vi "Meas Proc QWTB Multicore Start Servers.vi"(8 "error in":errorcluster, 11 "session in":T1={"adc"={"niScope"={"channel cfg"=[], "sessions"=[], "multi cards"=FALSE, "channels"=0, "type"=enum."n/a", "memory [B/chn]"=0, "ext. clock [Hz]"=0.0, "samples count"=0, "use streaming"=FALSE, "proc setup"={"packet size [smpl]"=0, "current timeout [s]"=0.0, "blk2blk timeout [s]"=0.0, "event time"=timestamp(0 s since 1904-01-01), "temp sampl T [s]"=0.0, "data queue"=refnum, "stop notifier"=refnum, "proc ref"=refnum}, "sample width [B]"=0, "ranges [V]"=[], "trigger setup"={"coupling"=1, "level [V]"=0.0, "slope"=0, "mode"=enum."Immediate"}, "fs [Hz]"=0.0, "bitres [bit]"=0, "clock source"=enum."VAL_NO_SOURCE"}, "3458A"={"channels"=[], "sync unit"={"VISA"="", "type"=enum."Picotest U6200A"}, "awg unit"={"type"=enum."Agilent 331xxA to 332xxA", "VISA"="", "enable 10MHz ref"=FALSE}, "sync mode"=enum."MASTER-SLAVE, MASTER clocked by TIMER", "streaming mode"=FALSE, "idn mode"=enum."Auto", "sampling mode"=enum."DCV", "Ts [s]"=0.0, "sample memory [B]"=0, "proc setup"={"channel id"=0, "packet size [smpl]"=0, "current timeout [s]"=0.0, "blk2blk timeout [s]"=0.0, "event time"=timestamp(0 s since 1904-01-01), "stop notifier"=refnum, "data queues"=[], "proc refs"=[], "bus semaphore"=refnum}, "sample size [B]"=0, "sample count"=0, "aux data"={"channel id"=0, "valid?"=[], "gain [V]"=[], "timestamp [s]"=[], "Ts [s]"=0.0, "abs timestamp"=timestamp(0 s since 1904-01-01), "t [deg C]"=[], "multiplex timestamp [s]"=-1.0, "only multiplex?"=FALSE, "multiplex smpl offset"=0}, "ranges [V]"=[], "aperture [s]"=0.0, "LEVEL trigger"={"edge"=enum."POS", "level [V]"=0.0, "coupling"=enum."DC"}, "trigger mode"=enum."AUTO", "measure temp.?"=FALSE, "disp mesages"=[], "shared bus?"=FALSE, "disable display?"=FALSE, "aper mode"=enum."Manual", "aper rules"=[], "multiplex"={"cycles"=0, "delay [s]"=0.0, "enabled"=FALSE, "overhead [s]"=1.0, "tot smpls"=0}}, "dsdll"={"dsdll"={"dsdll path"=path "", "dsdll handle"=[], "output devices"=[], "capture devices"=[]}, "channels"=0, "device id"=0, "channel idns"=[], "proc setup"={"packet size [smpl]"=0, "current timeout [s]"=0.0, "blk2blk timeout [s]"=0.0, "event time"=timestamp(0 s since 1904-01-01), "data queue"=refnum, "stop notifier"=refnum, "proc ref"=refnum}, "samples count"=0, "fs [Hz]"=0.0}, "type"=enum."niScope", "channel idn str"=[], "aux instr idn str"=[], "modified?"=FALSE, "simadc"={"channels"=[], "range [V]"=0.0, "Ts step [s]"=0.0, "time [s]"=0.0, "fs [Hz]"=0.0, "count"=0, "smpl offset"=0, "set count"=0, "bit res"=0}, "force rst?"=FALSE, "exit mode"=enum."Immediate reset", "exit dly"=0.0, "exit tmr"=timestamp(0 s since 1904-01-01), "busy?"=FALSE, "accessed?"=FALSE, "multiplex"={"Type"=enum."Dummy", "gen com ssn"={"visa"="", "primary"=enum."None", "secondary"=enum."None", "channels"=[]}, "delay before [s]"=0.0, "delay post [s]"=0.0, "sequence"=[], "enabled"=FALSE, "ref timestamp [s]"=0.0, "idn string"="", "dev niScope"="", "niScope idx"=0}}, "sequence"=[], "sequence setup"={"group setups"=[], "average cycles"=0, "range mode"=enum."Keep defaults", "fs mode"=enum."Frequency", "rng even"=0.0, "rng odd"=0.0, "folder"=path "", "name base"="", "meas id"=0, "settle [s]"=0.0, "comment"=""}, "golpi"=refnum, "processing setup"={"mode"=enum."Raw", "call after avgs?"=FALSE, "calculate?"=FALSE, "raw mode"={"command"="", "result mode"=enum."Display console output (only Octave)", "res variable"=""}, "QWTB"={"QWTB path"=path "", "alg filter path"="", "alg ids"=[], "alg parameters"=[], "parsed parameters"=[], "selected alg id"="", "selected unc mode"=enum."None", "qwtb mcc"=100, "qwtb timeout"=90, "qwtb covg"=95.0, "qwtb ofs"=0, "qwtb lim data"=0, "multicore"={"jobs folder"=path "", "cores"=0, "max jobs"=0, "mode"=enum."Singlecore"}, "unc once?"=FALSE, "qwtb tstemp"=enum."Enabled (default)", "octave reset"=FALSE}}, "corrections"={"transducers"={"channels"=[], "last path"=path ""}, "digitizer"={"last path"=path "", "channel paths"=[], "channel idns"=[], "correction name"="", "channel names"=[], "folders to copy"=[], "channel valid"=[], "correction path"=path "", "correction rel path"="", "rel folders to copy"=[]}}, "assist cfg"={"P"=0, "Q"=0, "rel shift"=0.0, "ref freq"=0.0, "min fs"=0.0, "max fs tol"=0.0, "min int"=0.0, "max int"=0.0, "max err"=0.0, "max timeout"=0.0}} {"corrections"."transducers"."channels"."Phase index" min=1 step=1; "adc"."3458A"."channels"."Range [Vpk]" min=0.0; "adc"."niScope"."trigger setup"."level [V]" format="%.2f"; "adc"."niScope"."trigger setup"."coupling" items=["AC"=0, "DC"=1, "HF Reject"=3, "LF Reject"=4, "AC Plus HF Reject"=1001]; "adc"."niScope"."channel cfg"."Range [Vpk]" min=0.0; "adc"."niScope"."channel cfg"."Channel" min=0}) -> (0 "error out":errorcluster, 3 "session out":T1={"adc"={"niScope"={"channel cfg"=[], "sessions"=[], "multi cards"=FALSE, "channels"=0, "type"=enum."n/a", "memory [B/chn]"=0, "ext. clock [Hz]"=0.0, "samples count"=0, "use streaming"=FALSE, "proc setup"={"packet size [smpl]"=0, "current timeout [s]"=0.0, "blk2blk timeout [s]"=0.0, "event time"=timestamp(0 s since 1904-01-01), "temp sampl T [s]"=0.0, "data queue"=refnum, "stop notifier"=refnum, "proc ref"=refnum}, "sample width [B]"=0, "ranges [V]"=[], "trigger setup"={"coupling"=1, "level [V]"=0.0, "slope"=0, "mode"=enum."Immediate"}, "fs [Hz]"=0.0, "bitres [bit]"=0, "clock source"=enum."VAL_NO_SOURCE"}, "3458A"={"channels"=[], "sync unit"={"VISA"="", "type"=enum."Picotest U6200A"}, "awg unit"={"type"=enum."Agilent 331xxA to 332xxA", "VISA"="", "enable 10MHz ref"=FALSE}, "sync mode"=enum."MASTER-SLAVE, MASTER clocked by TIMER", "streaming mode"=FALSE, "idn mode"=enum."Auto", "sampling mode"=enum."DCV", "Ts [s]"=0.0, "sample memory [B]"=0, "proc setup"={"channel id"=0, "packet size [smpl]"=0, "current timeout [s]"=0.0, "blk2blk timeout [s]"=0.0, "event time"=timestamp(0 s since 1904-01-01), "stop notifier"=refnum, "data queues"=[], "proc refs"=[], "bus semaphore"=refnum}, "sample size [B]"=0, "sample count"=0, "aux data"={"channel id"=0, "valid?"=[], "gain [V]"=[], "timestamp [s]"=[], "Ts [s]"=0.0, "abs timestamp"=timestamp(0 s since 1904-01-01), "t [deg C]"=[], "multiplex timestamp [s]"=-1.0, "only multiplex?"=FALSE, "multiplex smpl offset"=0}, "ranges [V]"=[], "aperture [s]"=0.0, "LEVEL trigger"={"edge"=enum."POS", "level [V]"=0.0, "coupling"=enum."DC"}, "trigger mode"=enum."AUTO", "measure temp.?"=FALSE, "disp mesages"=[], "shared bus?"=FALSE, "disable display?"=FALSE, "aper mode"=enum."Manual", "aper rules"=[], "multiplex"={"cycles"=0, "delay [s]"=0.0, "enabled"=FALSE, "overhead [s]"=1.0, "tot smpls"=0}}, "dsdll"={"dsdll"={"dsdll path"=path "", "dsdll handle"=[], "output devices"=[], "capture devices"=[]}, "channels"=0, "device id"=0, "channel idns"=[], "proc setup"={"packet size [smpl]"=0, "current timeout [s]"=0.0, "blk2blk timeout [s]"=0.0, "event time"=timestamp(0 s since 1904-01-01), "data queue"=refnum, "stop notifier"=refnum, "proc ref"=refnum}, "samples count"=0, "fs [Hz]"=0.0}, "type"=enum."niScope", "channel idn str"=[], "aux instr idn str"=[], "modified?"=FALSE, "simadc"={"channels"=[], "range [V]"=0.0, "Ts step [s]"=0.0, "time [s]"=0.0, "fs [Hz]"=0.0, "count"=0, "smpl offset"=0, "set count"=0, "bit res"=0}, "force rst?"=FALSE, "exit mode"=enum."Immediate reset", "exit dly"=0.0, "exit tmr"=timestamp(0 s since 1904-01-01), "busy?"=FALSE, "accessed?"=FALSE, "multiplex"={"Type"=enum."Dummy", "gen com ssn"={"visa"="", "primary"=enum."None", "secondary"=enum."None", "channels"=[]}, "delay before [s]"=0.0, "delay post [s]"=0.0, "sequence"=[], "enabled"=FALSE, "ref timestamp [s]"=0.0, "idn string"="", "dev niScope"="", "niScope idx"=0}}, "sequence"=[], "sequence setup"={"group setups"=[], "average cycles"=0, "range mode"=enum."Keep defaults", "fs mode"=enum."Frequency", "rng even"=0.0, "rng odd"=0.0, "folder"=path "", "name base"="", "meas id"=0, "settle [s]"=0.0, "comment"=""}, "golpi"=refnum, "processing setup"={"mode"=enum."Raw", "call after avgs?"=FALSE, "calculate?"=FALSE, "raw mode"={"command"="", "result mode"=enum."Display console output (only Octave)", "res variable"=""}, "QWTB"={"QWTB path"=path "", "alg filter path"="", "alg ids"=[], "alg parameters"=[], "parsed parameters"=[], "selected alg id"="", "selected unc mode"=enum."None", "qwtb mcc"=100, "qwtb timeout"=90, "qwtb covg"=95.0, "qwtb ofs"=0, "qwtb lim data"=0, "multicore"={"jobs folder"=path "", "cores"=0, "max jobs"=0, "mode"=enum."Singlecore"}, "unc once?"=FALSE, "qwtb tstemp"=enum."Enabled (default)", "octave reset"=FALSE}}, "corrections"={"transducers"={"channels"=[], "last path"=path ""}, "digitizer"={"last path"=path "", "channel paths"=[], "channel idns"=[], "correction name"="", "channel names"=[], "folders to copy"=[], "channel valid"=[], "correction path"=path "", "correction rel path"="", "rel folders to copy"=[]}}, "assist cfg"={"P"=0, "Q"=0, "rel shift"=0.0, "ref freq"=0.0, "min fs"=0.0, "max fs tol"=0.0, "min int"=0.0, "max int"=0.0, "max err"=0.0, "max timeout"=0.0}} {"corrections"."transducers"."channels"."Phase index" min=1 step=1; "adc"."3458A"."channels"."Range [Vpk]" min=0.0; "adc"."niScope"."trigger setup"."level [V]" format="%.2f"; "adc"."niScope"."trigger setup"."coupling" items=["AC"=0, "DC"=1, "HF Reject"=3, "LF Reject"=4, "AC Plus HF Reject"=1001]; "adc"."niScope"."channel cfg"."Range [Vpk]" min=0.0; "adc"."niScope"."channel cfg"."Channel" min=0})   [LabVIEW 2013]
doc: "Start multistation mode servers."
uses:
  Meas Session.ctl
  adc/ADC Session.ctl
  drivers/niScope/niScope Session.ctl
  drivers/niScope/niScope Virtual Channel Config.ctl
  drivers/niScope/niScope Virtual Channel Mode.ctl
  drivers/niScope/niScope Virtual Channel Input Z.ctl
  drivers/niScope/niScope Virtual Channel Coupling.ctl
  drivers/niScope/niScope Type.ctl
  drivers/niScope/niScope Digitizing Process Options.ctl
  drivers/niScope/niScope Data Packet.ctl
  drivers/niScope/niScope Trigger Setup.ctl
  <instrlib>/niScope/Controls/niScope trigger coupling.ctl
  <instrlib>/niScope/Controls/niScope trigger slope.ctl
  drivers/niScope/niScope Reference Clock.ctl
  drivers/DMM/3458A Digitizer Session.ctl
  drivers/DMM/3458A Virtual Channel Config.ctl
  drivers/Counter/Counter Session.ctl
  drivers/Counter/Counter Type.ctl
  drivers/AWG/AWG Session.ctl
  drivers/AWG/AWG Type.ctl
  drivers/DMM/3458A Sync Mode.ctl
  drivers/DMM/3458A Idn Mode.ctl
  drivers/DMM/3458A Digitizing Low Levels/Configure/Sampling Mode.ctl
  drivers/DMM/3458A Digitizing Process Options.ctl
  drivers/DMM/3458A Data Packet.ctl
  drivers/DMM/3458A Aux Record Data.ctl
  drivers/DMM/3458A Digitizing Low Levels/Configure/Level Setup.ctl
  drivers/DMM/3458A Digitizing Low Levels/Configure/First Sample Trigger.ctl
  drivers/DMM/3458A Aperture Selection Mode.ctl
  drivers/DMM/3458A Multiplexing Config.ctl
  drivers/dsdll/DSDLL Session.ctl
  drivers/dsdll/dsdll.lvlibp/dsdll_instance.ctl
  drivers/dsdll/dsdll.lvlibp/dsdll_device_record.ctl
  drivers/dsdll/DSDLL Process Config.ctl
  drivers/dsdll/DSDLL Data Packet.ctl
  adc/ADC Type.ctl
  drivers/simulated_adc/SimAdc Config.ctl
  drivers/simulated_adc/SimAdc Channel Cfg.ctl
  adc/ADC On Close Action.ctl
  adc/Multiplexer/MPX Session.ctl
  adc/Multiplexer/MPX Type.ctl
  drivers/Multiplexers/Generic COM/GCOMM Session.ctl
  drivers/Multiplexers/Generic COM/GCOMM Signal.ctl
  drivers/Multiplexers/Generic COM/GCOMM Virtual Channel.ctl
  drivers/Multiplexers/Generic COM/GCOMM Logic State.ctl
  Meas Sequence Item.ctl
  Meas Sampling Configuration.ctl
  adc/ADC Trig Config.ctl
  adc/ADC Trig Mode Source.ctl
  adc/ADC Trig Coupling.ctl
  adc/ADC Trig Slope.ctl
  Meas Proc QWTB Algorithm Parameter Data.ctl
  Meas Sequence Configuration.ctl
  Meas Range Mode.ctl
  Meas Sampling Rate Mode.ctl
  octave/golpi/mpc/golpi_session_ref.ctl
  octave/golpi/mpc/golpi_session.ctl
  octave/golpi/GOLPI Library.lvlibp/Public/GOLPI reference Type Def.ctl
  octave/golpi/GOLPI Library.lvlibp/LV Process source distribution/Pipe Handle.ctl
  Meas Process Config.ctl
  Meas Process Mode.ctl
  Meas Process Raw Config.ctl
  Meas Process Raw Result Mode.ctl
  Meas Proc QWTB Setup.ctl
  Meas Proc QWTB Uncertainty Mode.ctl
  Meas Proc QWTB Multicore Setup.ctl
  Meas Proc QWTB Multicore Type.ctl
  Meas Process Time Stamp Mode.ctl
  Corrections/Corr Setup.ctl
  Corrections/Corr Tranducer Item.ctl
  Corrections/Corr Digitizers.ctl
  Assist/Assist Panel Setup.ctl
  <vilib>/Utility/error.llb/Error Cluster From Error Code.vi
  <vilib>/ErrorRing/Error Ring.xnode
  octave/golpi/mpc/GOLPI Multi Process.lvlib
  octave/golpi/GOLPI Library.lvlibp
  drivers/niScope/niScope Virtual Digitizer.lvlib
  drivers/DMM/3458A Virtual Digitizer.lvlib
  drivers/Counter/Counter.lvlib
  drivers/AWG/AWG.lvlib
  drivers/DMM/3458A Digitizing Low Levels/3458A Digitizing Low Levels.lvlib
  drivers/dsdll/dsdll.lvlibp
  drivers/dsdll/DSDLL Virtual Digitizer.lvlib
  octave/golpi/GOLPI Library.lvlibp/LV Process source distribution/LV Process library.lvlib
panel:
  # "ADC:"
  # "ADC:"
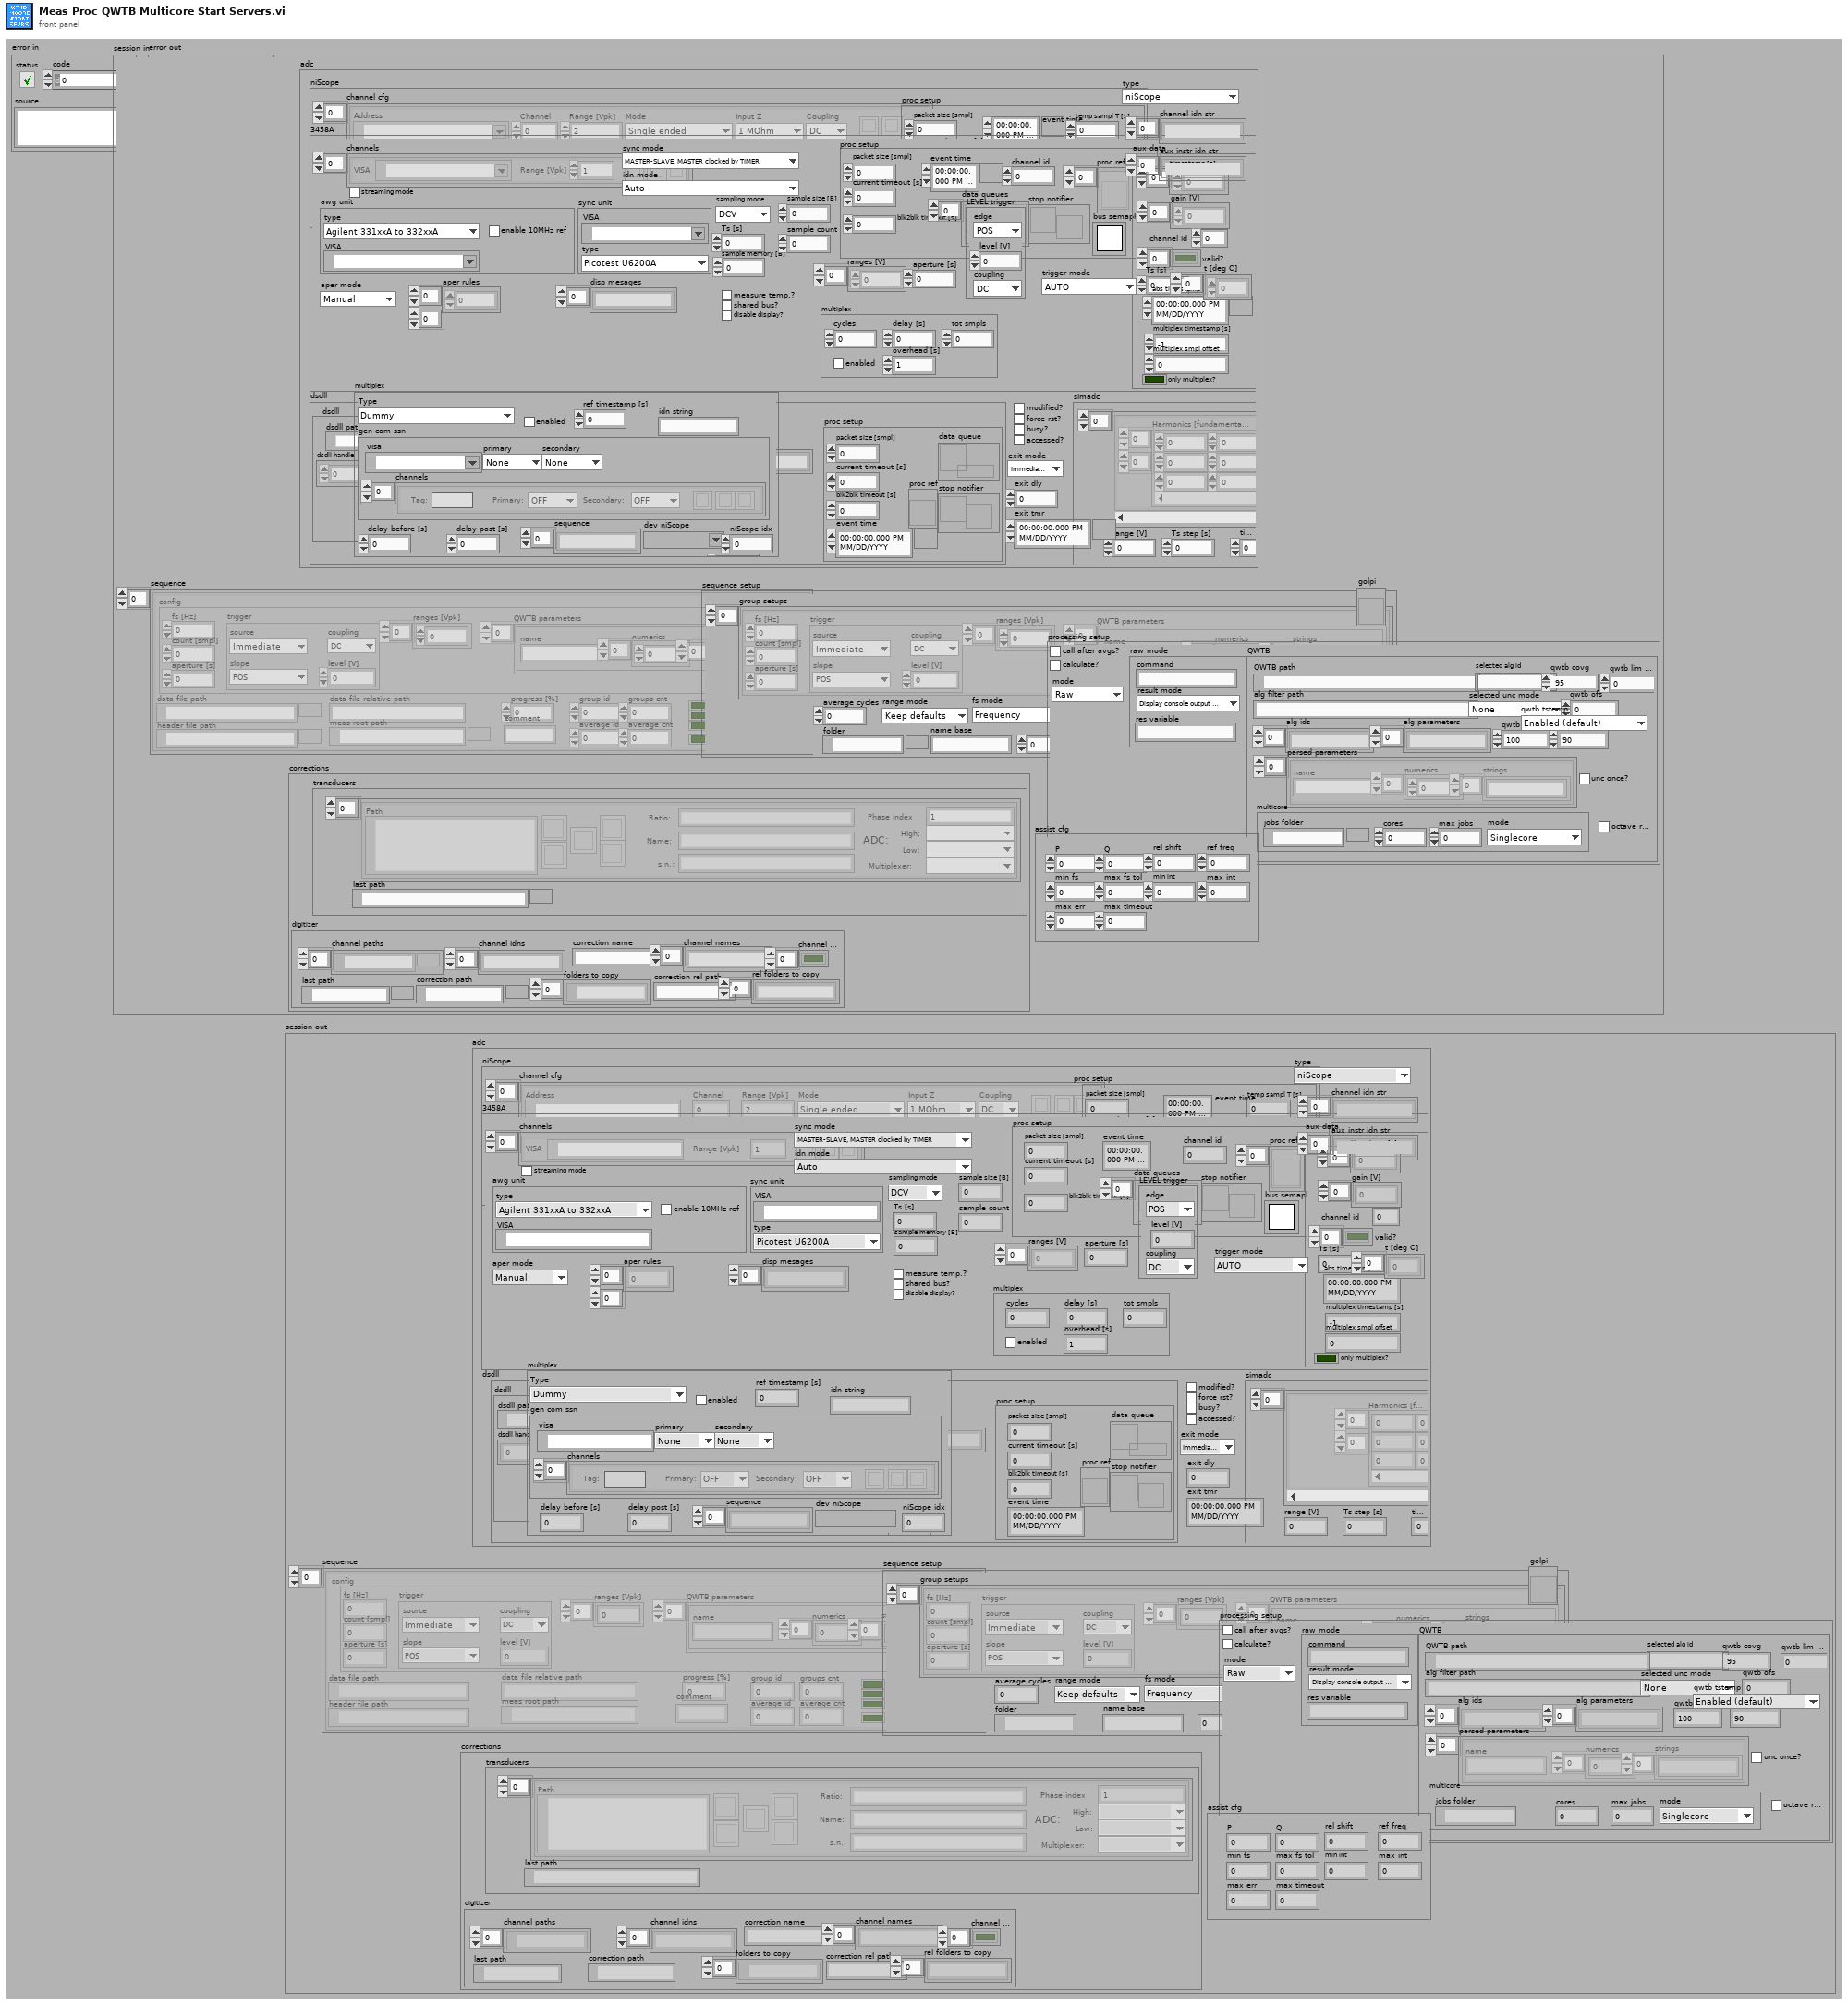
[diagram p1: front panel]
types:
  T1 = typedef "Meas Session.ctl" = cluster{"adc":T2, "sequence":T44[], "sequence setup":T51, "golpi":T54, "processing setup":T55, "corrections":T64, "assist cfg":T67}
  T2 = typedef "ADC Session.ctl" = cluster{"niScope":T3, "3458A":T14, "dsdll":T30, "type":T34, "channel idn str":string[], "aux instr idn str":string[], "modified?":bool, "simadc":T35, "force rst?":bool, "exit mode":T37, "exit dly":dbl, "exit tmr":timestamp, "busy?":bool, "accessed?":bool, "multiplex":T38}
  T3 = typedef "niScope Virtual Digitizer.lvlib/niScope Session.ctl" = cluster{"channel cfg":T4[], "sessions":refnum<k20>[], "multi cards":bool, "channels":i32, "type":T8, "memory [B/chn]":i32, "ext. clock [Hz]":dbl, "samples count":i64, "use streaming":bool, "proc setup":T9, "sample width [B]":i32, "ranges [V]":dbl[], "trigger setup":T10, "fs [Hz]":dbl, "bitres [bit]":i32, "clock source":T13}
  T4 = typedef "niScope Virtual Digitizer.lvlib/niScope Virtual Channel Config.ctl" = cluster{"Address":refnum<k15>, "Channel":i32, "Mode":T5, "Input Z":T6, "Coupling":T7, "Range [Vpk]":dbl, "btn clr":bool, "btn up":bool, "btn down":bool}
  T5 = typedef "niScope Virtual Digitizer.lvlib/niScope Virtual Channel Mode.ctl" = enum16{"Single ended", "Unbal. differential", "Differential"}
  T6 = typedef "niScope Virtual Digitizer.lvlib/niScope Virtual Channel Input Z.ctl" = enum16{"1 MOhm", "50 Ohm"}
  T7 = typedef "niScope Virtual Digitizer.lvlib/niScope Virtual Channel Coupling.ctl" = enum16{"AC", "DC", "GND"}
  T8 = typedef "niScope Virtual Digitizer.lvlib/niScope Type.ctl" = enum16{"n/a", "5922"}
  T9 = typedef "niScope Virtual Digitizer.lvlib/niScope Digitizing Process Options.ctl" = cluster{"packet size [smpl]":i64, "current timeout [s]":dbl, "blk2blk timeout [s]":dbl, "event time":timestamp, "temp sampl T [s]":dbl, "data queue":refnum<queue>, "stop notifier":refnum<notifier>, "proc ref":refnum<vi>}
  T10 = typedef "niScope Virtual Digitizer.lvlib/niScope Trigger Setup.ctl" = cluster{"coupling":T11, "level [V]":dbl, "slope":T12, "mode":enum16{"Immediate", "External", "Level"}}
  T11 = typedef "niScope trigger coupling.ctl" = u16
  T12 = typedef "niScope trigger slope.ctl" = i32
  T13 = typedef "niScope Virtual Digitizer.lvlib/niScope Reference Clock.ctl" = enum16{"VAL_NO_SOURCE", "VAL_CLK_IN", "VAL_PXI_CLOCK", "VAL_EXTERNAL"}
  T14 = typedef "3458A Virtual Digitizer.lvlib/3458A Digitizer Session.ctl" = cluster{"channels":T15[], "sync unit":T16, "awg unit":T18, "sync mode":T20, "streaming mode":bool, "idn mode":T21, "sampling mode":T22, "Ts [s]":dbl, "sample memory [B]":i32, "proc setup":T23, "sample size [B]":i32, "sample count":i32, "aux data":T25, "ranges [V]":dbl[], "aperture [s]":dbl, "LEVEL trigger":T26, "trigger mode":T27, "measure temp.?":bool, "disp mesages":string[], "shared bus?":bool, "disable display?":bool, "aper mode":T28, "aper rules":dbl[][], "multiplex":T29}
  T15 = typedef "3458A Virtual Digitizer.lvlib/3458A Virtual Channel Config.ctl" = cluster{"VISA":refnum<visa-resource-name>, "Range [Vpk]":dbl, "btn clr":bool, "btn up":bool, "btn down":bool}
  T16 = typedef "Counter.lvlib/Counter Session.ctl" = cluster{"VISA":refnum<visa-resource-name>, "type":T17}
  T17 = typedef "Counter.lvlib/Counter Type.ctl" = enum16{"Picotest U6200A", "dummy"}
  T18 = typedef "AWG.lvlib/AWG Session.ctl" = cluster{"type":T19, "VISA":refnum<visa-resource-name>, "enable 10MHz ref":bool}
  T19 = typedef "AWG.lvlib/AWG Type.ctl" = enum16{"Agilent 331xxA to 332xxA", "Agilent 335xxA to 336xxA", "Tektronix AFG3101C", "dummy"}
  T20 = typedef "3458A Virtual Digitizer.lvlib/3458A Sync Mode.ctl" = enum16{"MASTER-SLAVE, MASTER clocked by TIMER", "MASTER-SLAVE, MASTER clocked by AWG", "ALL clocked by AWG", "MASTER-SLAVE, ALL clocked by TIMER", "ALL clocked by AWG with DFLL"}
  T21 = typedef "3458A Virtual Digitizer.lvlib/3458A Idn Mode.ctl" = enum16{"Auto", "Sequential (chn A, chn B, ...)", "From calibration string"}
  T22 = typedef "3458A Virtual Digitizer.lvlib/3458A Digitizing Low Levels.lvlib/Sampling Mode.ctl" = enum16{"DCV", "DSDC", "DSAC"}
  T23 = typedef "3458A Virtual Digitizer.lvlib/3458A Digitizing Process Options.ctl" = cluster{"channel id":i32, "packet size [smpl]":i32, "current timeout [s]":dbl, "blk2blk timeout [s]":dbl, "event time":timestamp, "stop notifier":refnum<notifier>, "data queues":refnum<queue>[], "proc refs":refnum<vi>[], "bus semaphore":T24}
  T24 = typedef "Semaphore RefNum" = refnum<k1>
  T25 = typedef "3458A Virtual Digitizer.lvlib/3458A Aux Record Data.ctl" = cluster{"channel id":i32, "valid?":bool[], "gain [V]":dbl[], "timestamp [s]":dbl[], "Ts [s]":dbl, "abs timestamp":timestamp, "t [deg C]":dbl[], "multiplex timestamp [s]":dbl, "only multiplex?":bool, "multiplex smpl offset":i64}
  T26 = typedef "3458A Virtual Digitizer.lvlib/3458A Digitizing Low Levels.lvlib/Level Setup.ctl" = cluster{"edge":enum16{"POS", "NEG"}, "level [V]":dbl, "coupling":enum16{"DC", "AC"}}
  T27 = typedef "3458A Virtual Digitizer.lvlib/3458A Digitizing Low Levels.lvlib/First Sample Trigger.ctl" = enum16{"AUTO", "EXT", "SYN", "SGL", "HOLD", "LEVEL"}
  T28 = typedef "3458A Virtual Digitizer.lvlib/3458A Aperture Selection Mode.ctl" = enum16{"Manual", "Maximum", "Table"}
  T29 = typedef "3458A Multiplexing Config.ctl" = cluster{"cycles":i32, "delay [s]":dbl, "enabled":bool, "overhead [s]":dbl, "tot smpls":i64}
  T30 = typedef "DSDLL Virtual Digitizer.lvlib/DSDLL Session.ctl" = cluster{"dsdll":T31, "channels":i32, "device id":i32, "channel idns":string[], "proc setup":T33, "samples count":i32, "fs [Hz]":dbl}
  T31 = typedef "dsdll.lvlibp/dsdll_instance.ctl" = cluster{"dsdll path":path, "dsdll handle":u8[], "output devices":T32[], "capture devices":T32[]}
  T32 = typedef "dsdll.lvlibp/dsdll_device_record.ctl" = cluster{"guid":u8[], "name":string}
  T33 = typedef "DSDLL Virtual Digitizer.lvlib/DSDLL Process Config.ctl" = cluster{"packet size [smpl]":i32, "current timeout [s]":dbl, "blk2blk timeout [s]":dbl, "event time":timestamp, "data queue":refnum<queue>, "stop notifier":refnum<notifier>, "proc ref":refnum<vi>}
  T34 = typedef "ADC Type.ctl" = enum16{"niScope", "3458A", "DirectSound DLL", "dummy"}
  T35 = typedef "SimAdc Config.ctl" = cluster{"channels":T36[], "range [V]":dbl, "Ts step [s]":dbl, "time [s]":dbl, "fs [Hz]":dbl, "count":i64, "smpl offset":i64, "set count":i64, "bit res":i32}
  T36 = typedef "SimAdc Channel Cfg.ctl" = cluster{"harmonics":dbl[][], "btn clear":bool, "noise":dbl, "fundamental [Hz]":dbl}
  T37 = typedef "ADC On Close Action.ctl" = enum16{"Immediate reset", "Delayed reset"}
  T38 = typedef "MPX Session.ctl" = cluster{"Type":T39, "gen com ssn":T40, "delay before [s]":dbl, "delay post [s]":dbl, "sequence":string[], "enabled":bool, "ref timestamp [s]":dbl, "idn string":string, "dev niScope":refnum<k15>, "niScope idx":i32}
  T39 = typedef "MPX Type.ctl" = enum16{"Dummy", "Generic - COM port", "Generic - niScope PFI"}
  T40 = typedef "GCOMM Session.ctl" = cluster{"visa":refnum<visa-resource-name>, "primary":T41, "secondary":T41, "channels":T42[]}
  T41 = typedef "GCOMM Signal.ctl" = enum16{"None", "DTR", "RTS"}
  T42 = typedef "GCOMM Virtual Channel.ctl" = cluster{"Primary:":T43, "Secondary:":T43, "btn clr":bool, "btn up":bool, "btn down":bool, "Tag:":string}
  T43 = typedef "GCOMM Logic State.ctl" = enum16{"OFF", "ON"}
  T44 = typedef "Meas Sequence Item.ctl" = cluster{"config":T45, "data file path":path, "header file path":path, "group id":i32, "average id":i32, "group done?":bool, "adc modified?":bool, "source modified?":bool, "progress [%]":dbl, "groups cnt":i32, "average cnt":i32, "data file relative path":string, "meas root path":path, "calculate?":bool, "comment":string}
  T45 = typedef "Meas Sampling Configuration.ctl" = cluster{"fs [Hz]":dbl, "count [smpl]":i64, "aperture [s]":dbl, "trigger":T46, "ranges [Vpk]":dbl[], "QWTB parameters":T50[]}
  T46 = typedef "ADC Trig Config.ctl" = cluster{"source":T47, "level [V]":dbl, "coupling":T48, "slope":T49}
  T47 = typedef "ADC Trig Mode Source.ctl" = enum16{"Immediate", "External", "Level"}
  T48 = typedef "ADC Trig Coupling.ctl" = enum16{"DC", "AC"}
  T49 = typedef "ADC Trig Slope.ctl" = enum16{"POS", "NEG"}
  T50 = typedef "Meas Proc QWTB Algorithm Parameter Data.ctl" = cluster{"name":string, "numerics":dbl[], "strings":string[]}
  T51 = typedef "Meas Sequence Configuration.ctl" = cluster{"group setups":T45[], "average cycles":i32, "range mode":T52, "fs mode":T53, "rng even":dbl, "rng odd":dbl, "folder":path, "name base":string, "meas id":i32, "settle [s]":dbl, "comment":string}
  T52 = typedef "Meas Range Mode.ctl" = enum16{"Keep defaults", "Set All channels", "Set Odd and Even channels"}
  T53 = typedef "Meas Sampling Rate Mode.ctl" = enum16{"Frequency", "Period"}
  T54 = typedef "GOLPI Multi Process.lvlib/golpi_session_ref.ctl" = refnum<vi>
  T55 = typedef "Meas Process Config.ctl" = cluster{"mode":T56, "call after avgs?":bool, "calculate?":bool, "raw mode":T57, "QWTB":T59}
  T56 = typedef "Meas Process Mode.ctl" = enum16{"Raw", "QWTB"}
  T57 = typedef "Meas Process Raw Config.ctl" = cluster{"command":string, "result mode":T58, "res variable":string}
  T58 = typedef "Meas Process Raw Result Mode.ctl" = enum16{"Display console output (only Octave)", "Display string variable", "Display result file %respath%"}
  T59 = typedef "Meas Proc QWTB Setup.ctl" = cluster{"QWTB path":path, "alg filter path":string, "alg ids":string[], "alg parameters":string[], "parsed parameters":T50[], "selected alg id":string, "selected unc mode":T60, "qwtb mcc":i32, "qwtb timeout":i32, "qwtb covg":dbl, "qwtb ofs":i64, "qwtb lim data":i64, "multicore":T61, "unc once?":bool, "qwtb tstemp":T63, "octave reset":bool}
  T60 = typedef "Meas Proc QWTB Uncertainty Mode.ctl" = enum16{"None", "GUF", "Monte Carlo"}
  T61 = typedef "Meas Proc QWTB Multicore Setup.ctl" = cluster{"jobs folder":path, "cores":i32, "max jobs":i32, "mode":T62}
  T62 = typedef "Meas Proc QWTB Multicore Type.ctl" = enum16{"Singlecore", "Multicore", "Multistation"}
  T63 = typedef "Meas Process Time Stamp Mode.ctl" = enum16{"Enabled (default)", "Disabled", "Relative to 1. record"}
  T64 = typedef "Corr Setup.ctl" = cluster{"transducers":cluster{"channels":T65[], "last path":path}, "digitizer":T66}
  T65 = typedef "Corr Tranducer Item.ctl" = cluster{"Path":path, "Ratio:":string, "Name:":string, "btn rem":bool, "btn up":bool, "btn down":bool, "s.n.:":string, "btn open":bool, "ratio o/i":dbl, "chn hi":u16, "chn lo":u16, "Phase index":i32, "btn edit":bool, "mpx chn":u16}
  T66 = typedef "Corr Digitizers.ctl" = cluster{"last path":path, "channel paths":path[], "channel idns":string[], "correction name":string, "channel names":string[], "folders to copy":path[], "channel valid":bool[], "correction path":path, "correction rel path":string, "rel folders to copy":string[]}
  T67 = typedef "Assist Panel Setup.ctl" = cluster{"P":i32, "Q":i32, "rel shift":dbl, "ref freq":dbl, "min fs":dbl, "max fs tol":dbl, "min int":dbl, "max int":dbl, "max err":dbl, "max timeout":dbl}
  T68 = typedef "GOLPI Library.lvlibp/GOLPI reference Type Def.ctl" = cluster{"pipe handle":T69, "fast read timeout [ms]":u32, "fast read settle time [ms]":u32, "fast read to multiple [ms]":u32, "max elements per input line":u32, "slow read timeout [ms]":u32, "stdin double format specifier":string, "max elements per stdout output column":u32, "console mode bitstream":bool, "bitstream first read timeout [ms]":u32, "bitstream read timeout [ms]":u32, "struct transfer possible":bool, "matlab mode":bool}
  T69 = typedef "GOLPI Library.lvlibp/LV Process library.lvlib/Pipe Handle.ctl" = cluster{"lv_proc.dll file path":path, "process instance handle":u32[], "debug mode":bool, "debug data":cluster{"time":timestamp, "stdin":bool, "data":string}[]}
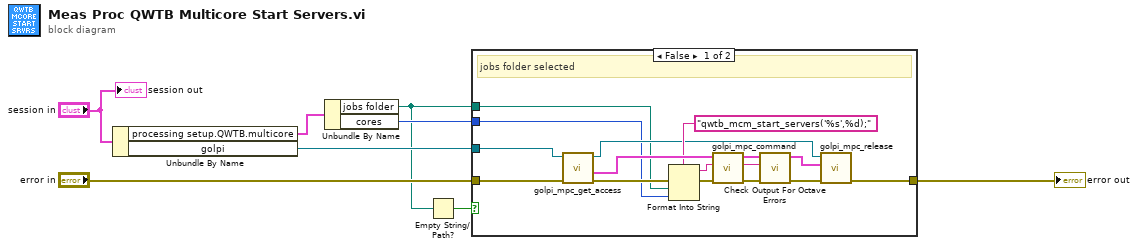
[diagram p0: block diagram]
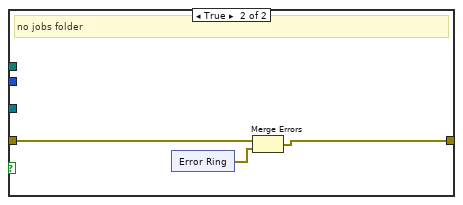
[diagram p2: hidden frame]
diagram:
  n1 = Unbundle By Name("session in") -> ("processing setup.QWTB.multicore"=w5:T61, "golpi"=w7:T54)
  n2 = Unbundle By Name(w5) -> ("jobs folder"=w2:path, "cores"=w4:i32)
  n3 = Empty String/Path?(string/path=w2) -> (empty?=w1:bool)
  n4 = case shown="False" w1 {
    tunnel: "error in" -> [w23 w26]
    tunnel: w7 -> [w21 _]
    tunnel: [w16 w25] -> w6
    tunnel: w4 -> [w14 _]
    tunnel: w2 -> [w9 _]
    frame False {
      # "jobs folder selected"
      n5 = call "golpi_mpc_get_access.vi"("error in"=w23, "golpi session ref"=w21) -> ("error out"=w19:errorcluster, "GOLPI ref out"=w22:T68, "golpi session ref out (copy)"=w17:T54)  [unwired: 4 in, 3 out]
      n6 = Format Into String(format string="qwtb_mcm_start_servers('%s',%d);" ("command"), error in=w19, w9, w14) -> (resulting string=w15:string, error out=w20:errorcluster)  [unwired: 1 in]
      n7 = call "golpi_mpc_command.vi"("error in"=w20, "command"=w15, "GOLPI ref in"=w22) -> ("error out"=w13:errorcluster, "read buffer"=w12:string, "GOLPI ref. out"=w10:T68)  [unwired: 6 in]
      n8 = call "Check Output For Octave Errors.vi"("error in"=w13, "read buffer"=w12) -> ("error out"=w11:errorcluster)  [unwired: 9 in]
      n9 = call "golpi_mpc_release.vi"("error in"=w11, "golpi ref or golpi session in"=w10, "golpi session ref"=w17) -> ("error out"=w16:errorcluster)  [unwired: 7 in, 1 out]
    }
    frame True {
      # "no jobs folder"
      n10 = xnode "Error Ring"() -> ("error out"=w24:errorcluster)
      n11 = Merge Errors(w26, w24) -> (w25:errorcluster)
    }
  }
  "error out" <- w6
  "session out" <- "session in"
